vi "Peek.vi"(8 "error in (no error)":errorcluster, 11 "Signaller in":refnum<class "Signaller.lvclass">) -> (0 "error out":errorcluster, 2 "Has signal":bool, 3 "Signaller out":refnum<class "Signaller.lvclass">)   [LabVIEW 2018, in "Signaller.lvclass"]
uses:
  Signaller.lvclass
  Signaller.lvclass/Signaller.ctl
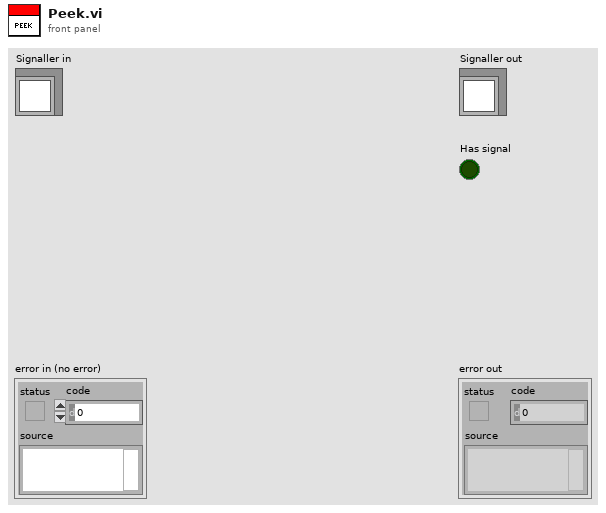
[diagram p1: front panel]
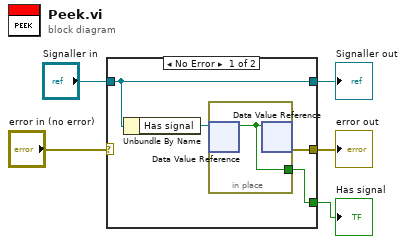
[diagram p0: block diagram]
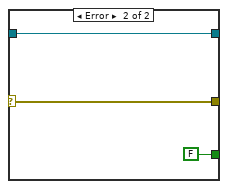
[diagram p2: hidden frame]
diagram:
  n1 = case shown="No Error" "error in (no error)" {
    selector: "error in (no error)" -> [_ w12]
    tunnel: [w7 w12] -> w4
    tunnel: [w9 w13] -> w2
    tunnel: "Signaller in" -> [w9 w13]
    tunnel: [w8 FALSE ("Boolean")] -> w1
    frame No Error {
      n2 = Unbundle By Name(w9) -> ("Has signal"=w6:refnum<data-value>)
      n3 = in-place {
        in-place-border: [w10] -> w8
        n4 = in-place-dvr #1(w6) -> (w10:bool)  [unwired: 1 out]
        n5 = in-place-dvr #1(w10) -> (w7:errorcluster)  [unwired: 1 out]
      }
    }
    frame Error {
    }
  }
  "error out" <- w4
  "Signaller out" <- w2
  "Has signal" <- w1
